vi "Create new save file.vi"(2 "Insert":string, 3 "Ext":string=".dat", 4 "Index In":dbl=1.0) -> (0 "Path Out":path, 1 "Index Out":dbl)   [LabVIEW 2014]
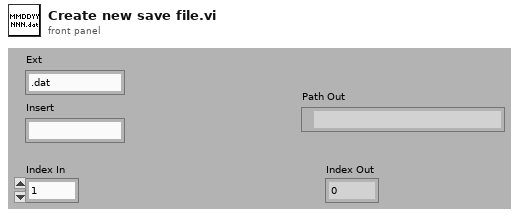
[diagram p1: front panel]
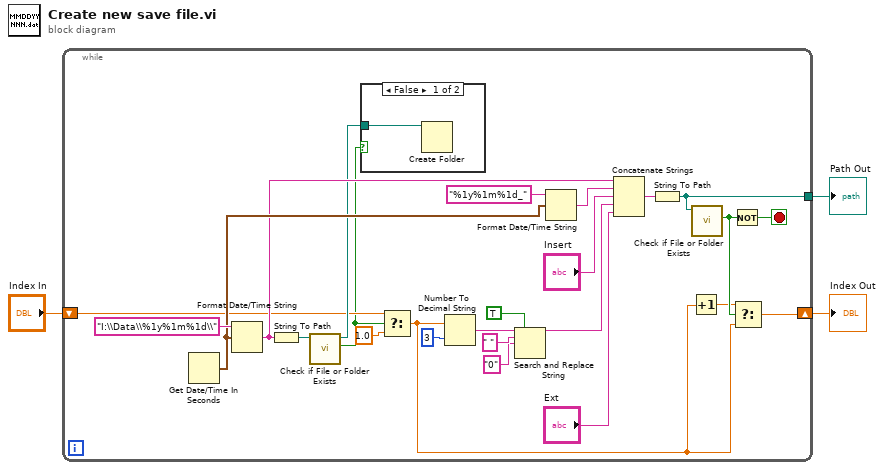
[diagram p0: block diagram]
diagram:
  n1 = while {
    tunnel: [w22] -> w2
    shift-right: [w20] -> w1
    shift-left: "Index In" -> [w7]
    stop <- w21 stop-if-true
    n2 = Get Date/Time In Seconds() -> (seconds since 1Jan1904=w14:timestamp)
    n3 = Format Date/Time String(time format string (%c)="I:\\Data\\%1y%1m%1d\\", seconds (now)=w14) -> (date/time string=w10:string)  [unwired: 1 out]
    n4 = String To Path(string=w10) -> (path=w9:path)
    n5 = call <vilib>:"Check if File or Folder Exists.vi"("path"=w9) -> ("file or folder exists?"=w5:bool, "dup path"=w8:path)  [unwired: 1 in, 8 out]
    n6 = case shown="False" w5 {
      tunnel: w8 -> [w29 _]
      frame False {
        n7 = Create Folder(path (use dialog)=w29) -> ()  [unwired: 1 in, 4 out]
      }
      frame True {
      }
    }
    n8 = Select(t=w7, s=w5, f=1.0) -> (s? t:f=w6:dbl)
    n9 = Number To Decimal String(number=w6, width (-)=i16 3) -> (decimal integer string=w24:string)
    n10 = Search and Replace String(replace all?=TRUE ("replace all? (F)"), input string=w24, search string=" ", replace string="0" ("replace string (\"\")")) -> (result string=w13:string)  [unwired: 1 in, 6 out]
    n11 = Format Date/Time String(time format string (%c)="%1y%1m%1d_", seconds (now)=w14) -> (date/time string=w27:string)  [unwired: 1 out]
    n12 = Concatenate Strings(w10, w27, "Insert", w13, "Ext") -> (w28:string)
    n13 = String To Path(string=w28) -> (path=w22:path)
    n14 = Increment(x=w6) -> (x+1=w18:dbl)
    n15 = call <vilib>:"Check if File or Folder Exists.vi"("path"=w22) -> ("file or folder exists?"=w19:bool)  [unwired: 1 in, 9 out]
    n16 = Not(x=w19) -> (.not. x?=w21:bool)
    n17 = Select(t=w18, s=w19, f=w6) -> (s? t:f=w20:dbl)
  }
  "Index Out" <- w1
  "Path Out" <- w2
